vi "receive_photon_buffer.vi"(8 "error in (no error)":errorcluster, 11 "tt20 in":refnum<class "tt20.lvclass">) -> (0 "error out":errorcluster, 2 "done":bool, 3 "tt20 out":refnum<class "tt20.lvclass">)   [LabVIEW 2015, in "tt20.lvclass"]
uses:
  tt20.lvclass
  tt20.lvclass/tt20.ctl
  C:/Users/MX-Microscope/Documents/LabVIEW Data/lvoop_campus_2018/Detector_Class/Swabian/time_tagger_vis/TTCSharp32.dll
  time_tagger_vis/TTCSharp32.dll
  tt20_buffer_tdef.ctl
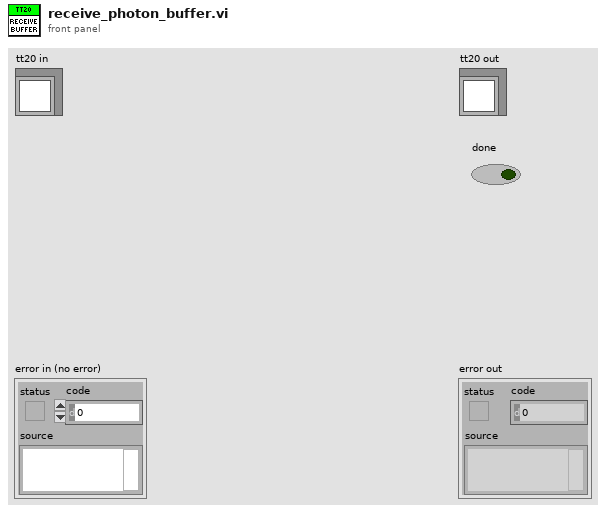
[diagram p1: front panel]
types:
  T1 = typedef "tt20_buffer_tdef.ctl" = cluster{"tagChannels":u32[], "tagTimestamps":i64[], "size":i32}
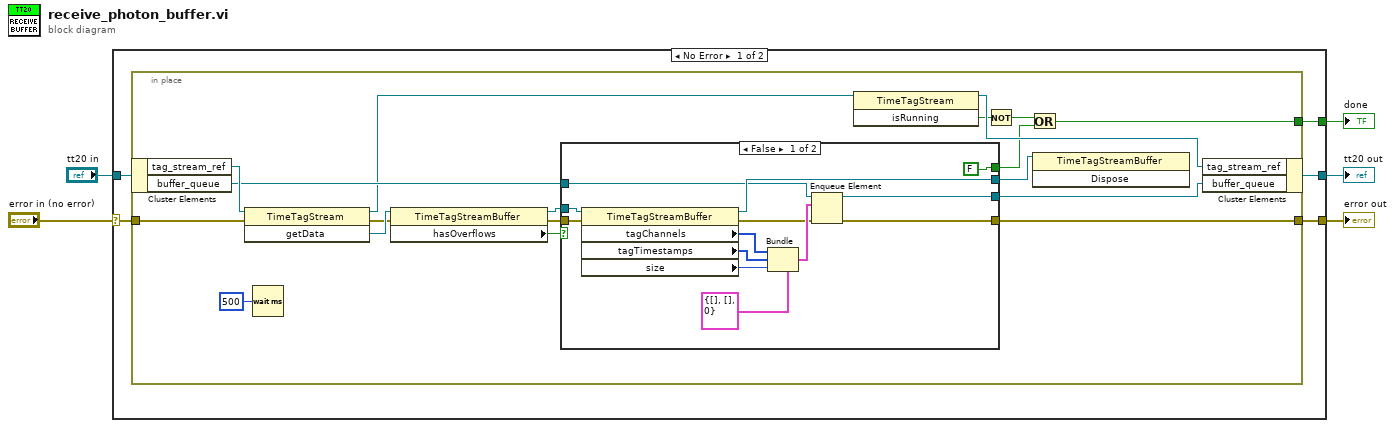
[diagram p0: block diagram]
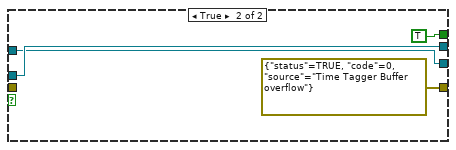
[diagram p2: hidden frame]
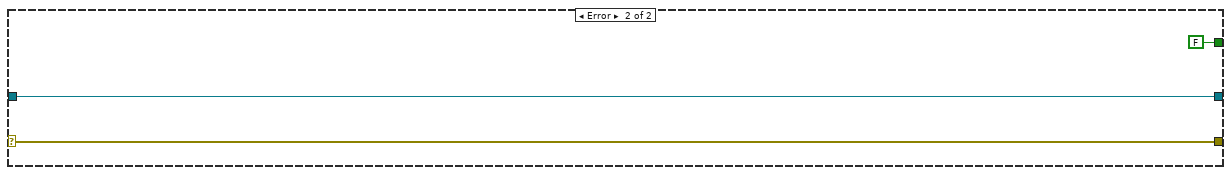
[diagram p3: hidden frame]
diagram:
  n1 = case shown="No Error" "error in (no error)" {
    selector: "error in (no error)" -> [w9 w47]
    tunnel: "tt20 in" -> [w10 w46]
    tunnel: [w8 w47] -> w3
    tunnel: [w7 w46] -> w2
    tunnel: [w6 FALSE] -> w1
    frame No Error {
      n2 = in-place {
        in-place-border: w9 -> [w27]
        in-place-border: [w16] -> w8
        in-place-border: [w14] -> w6
        n3 = in-place-cluster #1(w10) -> ("tag_stream_ref"=w28:refnum<k24>, "buffer_queue"=w20:refnum<queue>)
        n4 = invoke class="TimeTagStream" method="getData"(reference=w28, error in=w27) -> (reference out=w18:refnum<k24>, error out=w23:errorcluster, "getData"=w26:refnum<k24>)  [unwired: 1 in]
        n5 = Wait (ms)(milliseconds to wait=u32 500) -> ()  [unwired: 1 out]
        n6 = property class="TimeTagStreamBuffer"(reference=w26, error in=w23) -> (reference out=w25:refnum<k24>, error out=w21:errorcluster, "hasOverflows"=w24:bool)
        n7 = case shown="False" w24 {
          tunnel: w25 -> [w41 w45]
          tunnel: [w40 w45] -> w22
          tunnel: w21 -> [w39 _]
          tunnel: [w29 errorcluster {"status"=TRUE, "code"=0, "source"="Time Tagger Buffer overflow"} ("error out")] -> w16
          tunnel: [FALSE TRUE] -> w15
          tunnel: w20 -> [w32 w42]
          tunnel: [w31 w42] -> w19
          frame False {
            n8 = property class="TimeTagStreamBuffer"(reference=w41, error in=w39) -> (reference out=w40:refnum<k24>, error out=w30:errorcluster, "tagChannels"=w37:u32[], "tagTimestamps"=w36:i64[], "size"=w35:i32)
            n9 = Bundle(cluster=T1 {"tagChannels"=[], "tagTimestamps"=[], "size"=0} ("output cluster"), "tagChannels"=w37, "tagTimestamps"=w36, "size"=w35) -> (w33:T1)
            n10 = Enqueue Element(queue=w32, element=w33, error in (no error)=w30) -> (queue out=w31:refnum<queue>, error out=w29:errorcluster)  [unwired: 1 in, 1 out]
          }
          frame True {
          }
        }
        n11 = invoke class="TimeTagStream" method="isRunning"(reference=w18) -> (reference out=w17:refnum<k24>, "isRunning"=w13:bool)  [unwired: 2 in, 1 out]
        n12 = Not(x=w13) -> (.not. x?=w12:bool)
        n13 = Or(x=w12, y=w15) -> (x .or. y?=w14:bool)
        n14 = invoke class="TimeTagStreamBuffer" method="Dispose"(reference=w22) -> ()  [unwired: 2 in, 3 out]
        n15 = in-place-cluster #1("tag_stream_ref"=w17, "buffer_queue"=w19) -> (w7:refnum<class "tt20.lvclass">)
      }
    }
    frame Error {
    }
  }
  "error out" <- w3
  "tt20 out" <- w2
  "done" <- w1
